vi "Compare_values_Modify_Cost_f()-3.vi"(0 "[IN] Angles betwe\nen displacements":dbl[](array[numeric]), 1 "[IN] Array of displa\ncement differences":dbl[](array[numeric]), 2 "[IN] 3 Subsequent problem points in subtrack":bool, 3 "[IN] Cost function":i8[](array[numeric]), 5 "[IN] Reverse or not":bool[](array[boolean]), 9 "[IN] Areas \ndifferences":dbl[](array[numeric]), 11 "[IN] Statuses of points":i16[](array[numeric]), 12 "[IN] Additions to cost":i8[](array[numeric]), 13 "error IN":errorcluster) -> (4 "[OUT] Cost function":i8[](array[numeric]), 15 "error OUT":errorcluster)   [LabVIEW 2013]
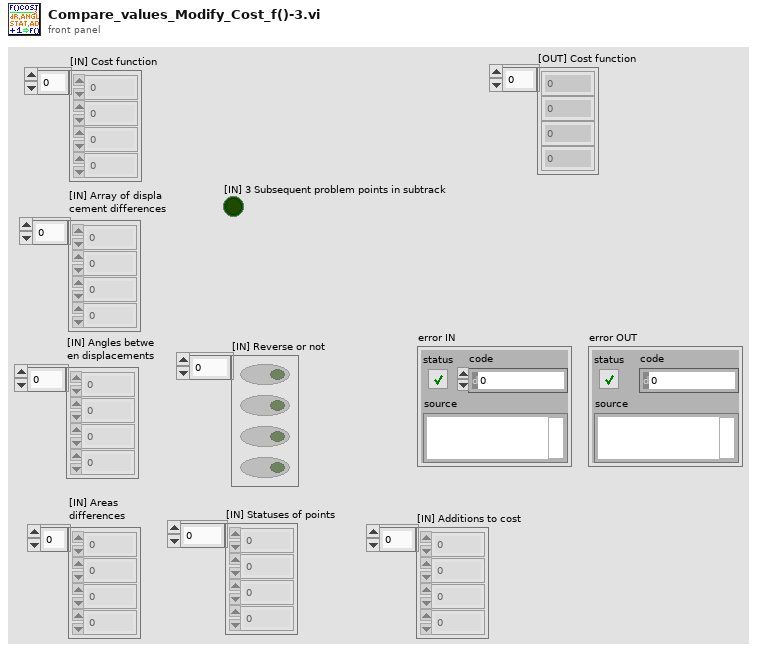
[diagram p1: front panel]
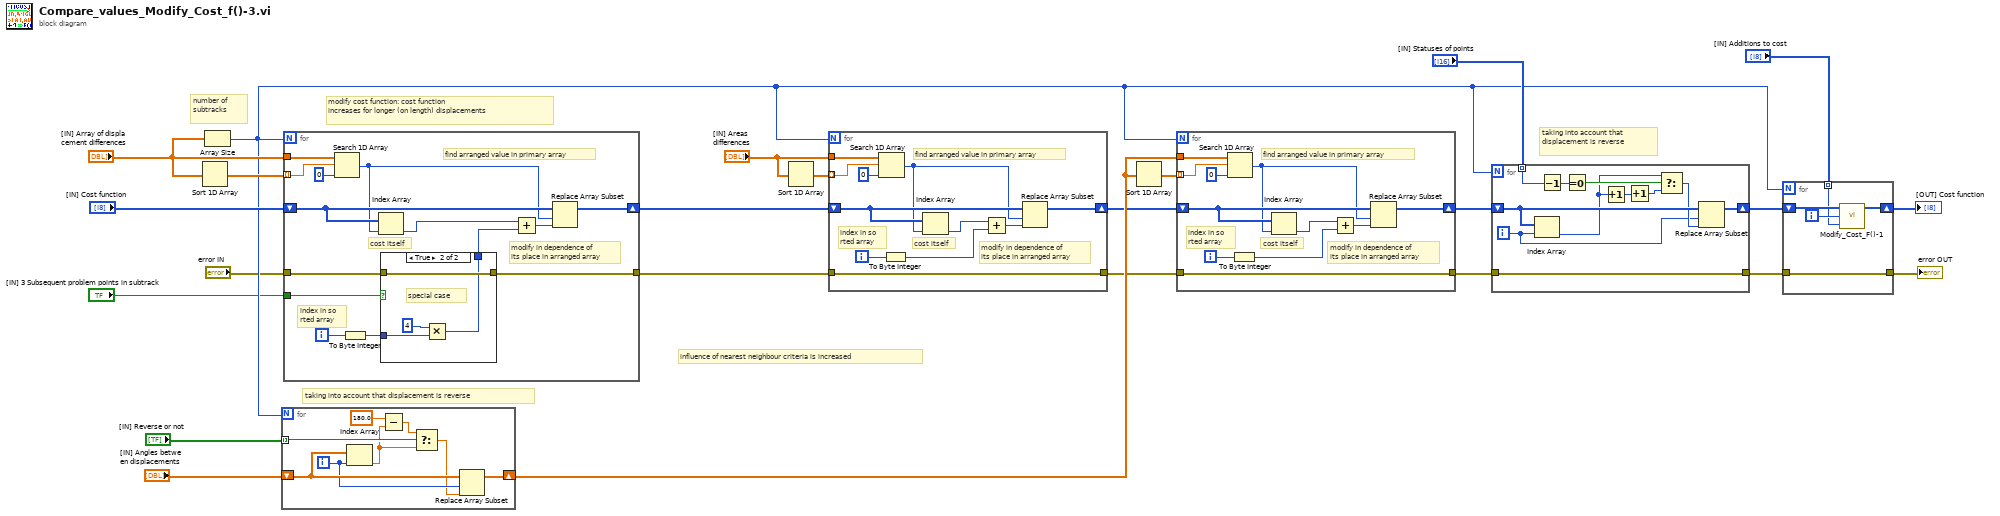
[diagram p0: block diagram]
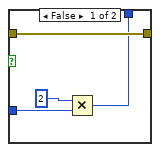
[diagram p2: hidden frame]
diagram:
  # "influence of nearest neighbour criteria is increased"
  # "taking into account that \ndisplacement is reverse"
  # "taking into account that displacement is reverse"
  # "modify cost function: cost function \nincreases for longer (on length) displacements"
  # "number of \nsubtracks"
  n1 = Sort 1D Array(array="[IN] Array of displa\ncement differences") -> (sorted array=w24:dbl[])
  n2 = Array Size(array="[IN] Array of displa\ncement differences") -> (size(s)=w11:i32)
  n3 = for {
    N: w11 -> [_]
    shift-right: [w25] -> w15
    shift-left: "[IN] Angles betwe\nen displacements" -> [w31]
    tunnel: "[IN] Reverse or not" -> [w32] mode=indexing
    i -> [w27]
    n4 = Index Array(array=w31, index=w27) -> (element=w29:dbl)
    n5 = Subtract(x=180.0, y=w29) -> (x-y=w28:dbl)
    n6 = Select(t=w28, s=w32, f=w29) -> (s? t:f=w26:dbl)
    n7 = Replace Array Subset(array=w31, new element=w26, index=w27) -> (w25:dbl[])
  }
  n8 = for {
    N: w11 -> [_]
    tunnel: w24 -> [w44] mode=indexing
    tunnel: "[IN] Array of displa\ncement differences" -> [w46]
    shift-right: [w38] -> w21
    shift-left: "[IN] Cost function" -> [w43]
    tunnel: "error IN" -> [w37]
    tunnel: [w36] -> w6
    tunnel: "[IN] 3 Subsequent problem points in subtrack" -> [w35]
    i -> [w39]
    # "modify in dependence of \nits place in arranged array"
    # "find arranged value in primary array"
    # "index in so\nrted array"
    # "cost itself"
    n9 = Search 1D Array(1D array=w46, element=w44, start index (0)=0) -> (index of element=w42:i32)
    n10 = To Byte Integer(number=w39) -> (8bit integer=w34:i8)
    n11 = Index Array(array=w43, index=w42) -> (element=w41:i8)
    n12 = case shown="True" w35 {
      tunnel: w37 -> [w50 w54]
      tunnel: [w50 w54] -> w36
      tunnel: w34 -> [w49 w53]
      tunnel: [w47 w51] -> w33
      frame False {
        n13 = Multiply(x=i8 2, y=w49) -> (x*y=w47:i8)
      }
      frame True {
        # "special case"
        n14 = Multiply(x=i8 4, y=w53) -> (x*y=w51:i8)
      }
    }
    n15 = Add(x=w41, y=w33) -> (x+y=w40:i8)
    n16 = Replace Array Subset(array=w43, new element=w40, index=w42) -> (w38:i8[])
  }
  n17 = Sort 1D Array(array="[IN] Areas \ndifferences") -> (sorted array=w19:dbl[])
  n18 = for {
    N: w11 -> [_]
    tunnel: w19 -> [w63] mode=indexing
    tunnel: "[IN] Areas \ndifferences" -> [w65]
    shift-right: [w56] -> w14
    shift-left: w21 -> [w62]
    tunnel: w6 -> [w55]
    tunnel: [w55] -> w5
    i -> [w58]
    # "modify in dependence of \nits place in arranged array"
    # "find arranged value in primary array"
    # "index in so\nrted array"
    # "cost itself"
    n19 = Search 1D Array(1D array=w65, element=w63, start index (0)=0) -> (index of element=w61:i32)
    n20 = To Byte Integer(number=w58) -> (8bit integer=w57:i8)
    n21 = Index Array(array=w62, index=w61) -> (element=w60:i8)
    n22 = Add(x=w60, y=w57) -> (x+y=w59:i8)
    n23 = Replace Array Subset(array=w62, new element=w59, index=w61) -> (w56:i8[])
  }
  n24 = Sort 1D Array(array=w15) -> (sorted array=w16:dbl[])
  n25 = for {
    N: w11 -> [_]
    tunnel: w16 -> [w74] mode=indexing
    tunnel: w15 -> [w76]
    shift-right: [w67] -> w13
    shift-left: w14 -> [w73]
    tunnel: w5 -> [w66]
    tunnel: [w66] -> w4
    i -> [w69]
    # "modify in dependence of \nits place in arranged array"
    # "find arranged value in primary array"
    # "index in so\nrted array"
    # "cost itself"
    n26 = Search 1D Array(1D array=w76, element=w74, start index (0)=0) -> (index of element=w72:i32)
    n27 = To Byte Integer(number=w69) -> (8bit integer=w68:i8)
    n28 = Index Array(array=w73, index=w72) -> (element=w71:i8)
    n29 = Add(x=w71, y=w68) -> (x+y=w70:i8)
    n30 = Replace Array Subset(array=w73, new element=w70, index=w72) -> (w67:i8[])
  }
  n31 = for {
    N: w11 -> [_]
    shift-right: [w78] -> w10
    shift-left: w13 -> [w87]
    tunnel: "[IN] Statuses of points" -> [w86] mode=indexing
    tunnel: w4 -> [w77]
    tunnel: [w77] -> w3
    i -> [w79]
    n32 = Index Array(array=w87, index=w79) -> (element=w83:i8)
    n33 = Decrement(x=w86) -> (x-1=w85:i16)
    n34 = Equal To 0?(x=w85) -> (x = 0?=w84:bool)
    n35 = Increment(x=w83) -> (x+1=w82:i8)
    n36 = Increment(x=w82) -> (x+1=w81:i8)
    n37 = Select(t=w83, s=w84, f=w81) -> (s? t:f=w80:i8)
    n38 = Replace Array Subset(array=w87, new element=w80, index=w79) -> (w78:i8[])
  }
  n39 = for {
    N: w11 -> [_]
    shift-right: [w89] -> w8
    shift-left: w10 -> [w92]
    tunnel: "[IN] Additions to cost" -> [w90] mode=indexing
    tunnel: w3 -> [w88]
    tunnel: [w88] -> w2
    i -> [w91]
    n40 = call "Modify_Cost_F()-1.vi"("[IN] Additions to cost"=w90, "[IN] Current Index"=w91, "[IN] Cost function"=w92) -> ("[OUT] Cost function"=w89:i8[])  [unwired: 2 in]
  }
  "[OUT] Cost function" <- w8
  "error OUT" <- w2
